vi "FLL Tournament Display.vi"() -> ()   [LabVIEW 2013]
uses:
  Team_List_Ctrl.ctl
  Team_Scores_And_Rankings_Array_Ctrl.ctl
  Round_And_Score_Ctrl.ctl
  Timer_Details_Ctrl.ctl
  <vilib>/httpClient/LabVIEWHTTPClient.lvlib
panel:
  out "Cancelled?":bool
  out "IP Address / Port":string
  in  "Scores Tab":enum32{"Page 1"}(tab)
  in  "Scores Box":i32(listbox)=3
  in  "Top Tab":enum32{"Page 1"}(tab)
  out "Main Logo Image":picture
  out "Powered By LabVIEW":picture
  out "FIRST LEGO League":picture
  out "Match Indicator":string
  out "Tournament Title String":string="2013 FIRST LEGO League Nature's Fury"
  out "TIMER":string="2 : 3 0"
  out "Top Sponsor Image":picture
  out "Mid Sponsor Image":picture
  out "Bottom Sponsor Image":picture
  out "Timer Properties":T1
  out "Consolidated Scores and Rankings":T3(array[cluster])
  out "Reported Scores and Rankings":T4
  out "Full Team List":T5[](array[typedef])
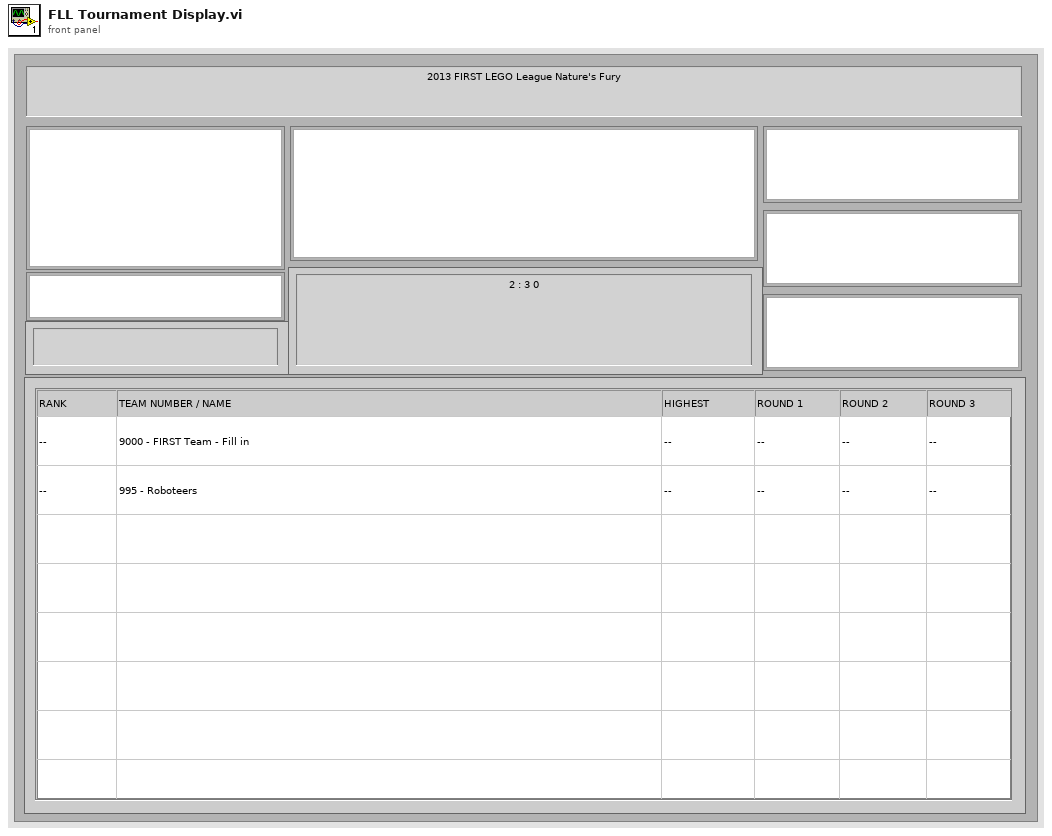
[diagram p1: front panel]
types:
  T1 = typedef "Timer_Details_Ctrl.ctl" = cluster{"TimeRemaining":string, "MatchPhase":string, "CurrentMatch":string, "Timer_Running":string}
  T2 = typedef "Round_And_Score_Ctrl.ctl" = cluster{"Score":string, "Round Number":string}
  T3 = cluster{"Rank":string, "Team Number":string, "Team Name":string, "Highest Score":string, "Scores":T2[]}[]
  T4 = typedef "Team_Scores_And_Rankings_Array_Ctrl.ctl" = cluster{"Rank":string, "Team Number":string, "Team Name":string, "Highest Score":string, "Scores":T2[]}[]
  T5 = typedef "Team_List_Ctrl.ctl" = cluster{"Team Name":string, "Team Number":string}
  T6 = typedef "LabVIEWHTTPClient.lvlib/ClientHandle.ctl" = refnum<k1>
  T7 = typedef "Team_List_Array_Ctrl.ctl" = T5[]
  T8 = cluster{"[0]":string, "[1]":string, "[2]":string, "[3]":string}
  T9 = enum32{"Invalid", "Standard", "Closed", "Hidden", "Minimized", "Maximized"}
  T10 = enum32{"invalid app kind", "Development System", "Run Time System", "Student Edition", "Embedded LabVIEW", "Evaluation", "Custom"}
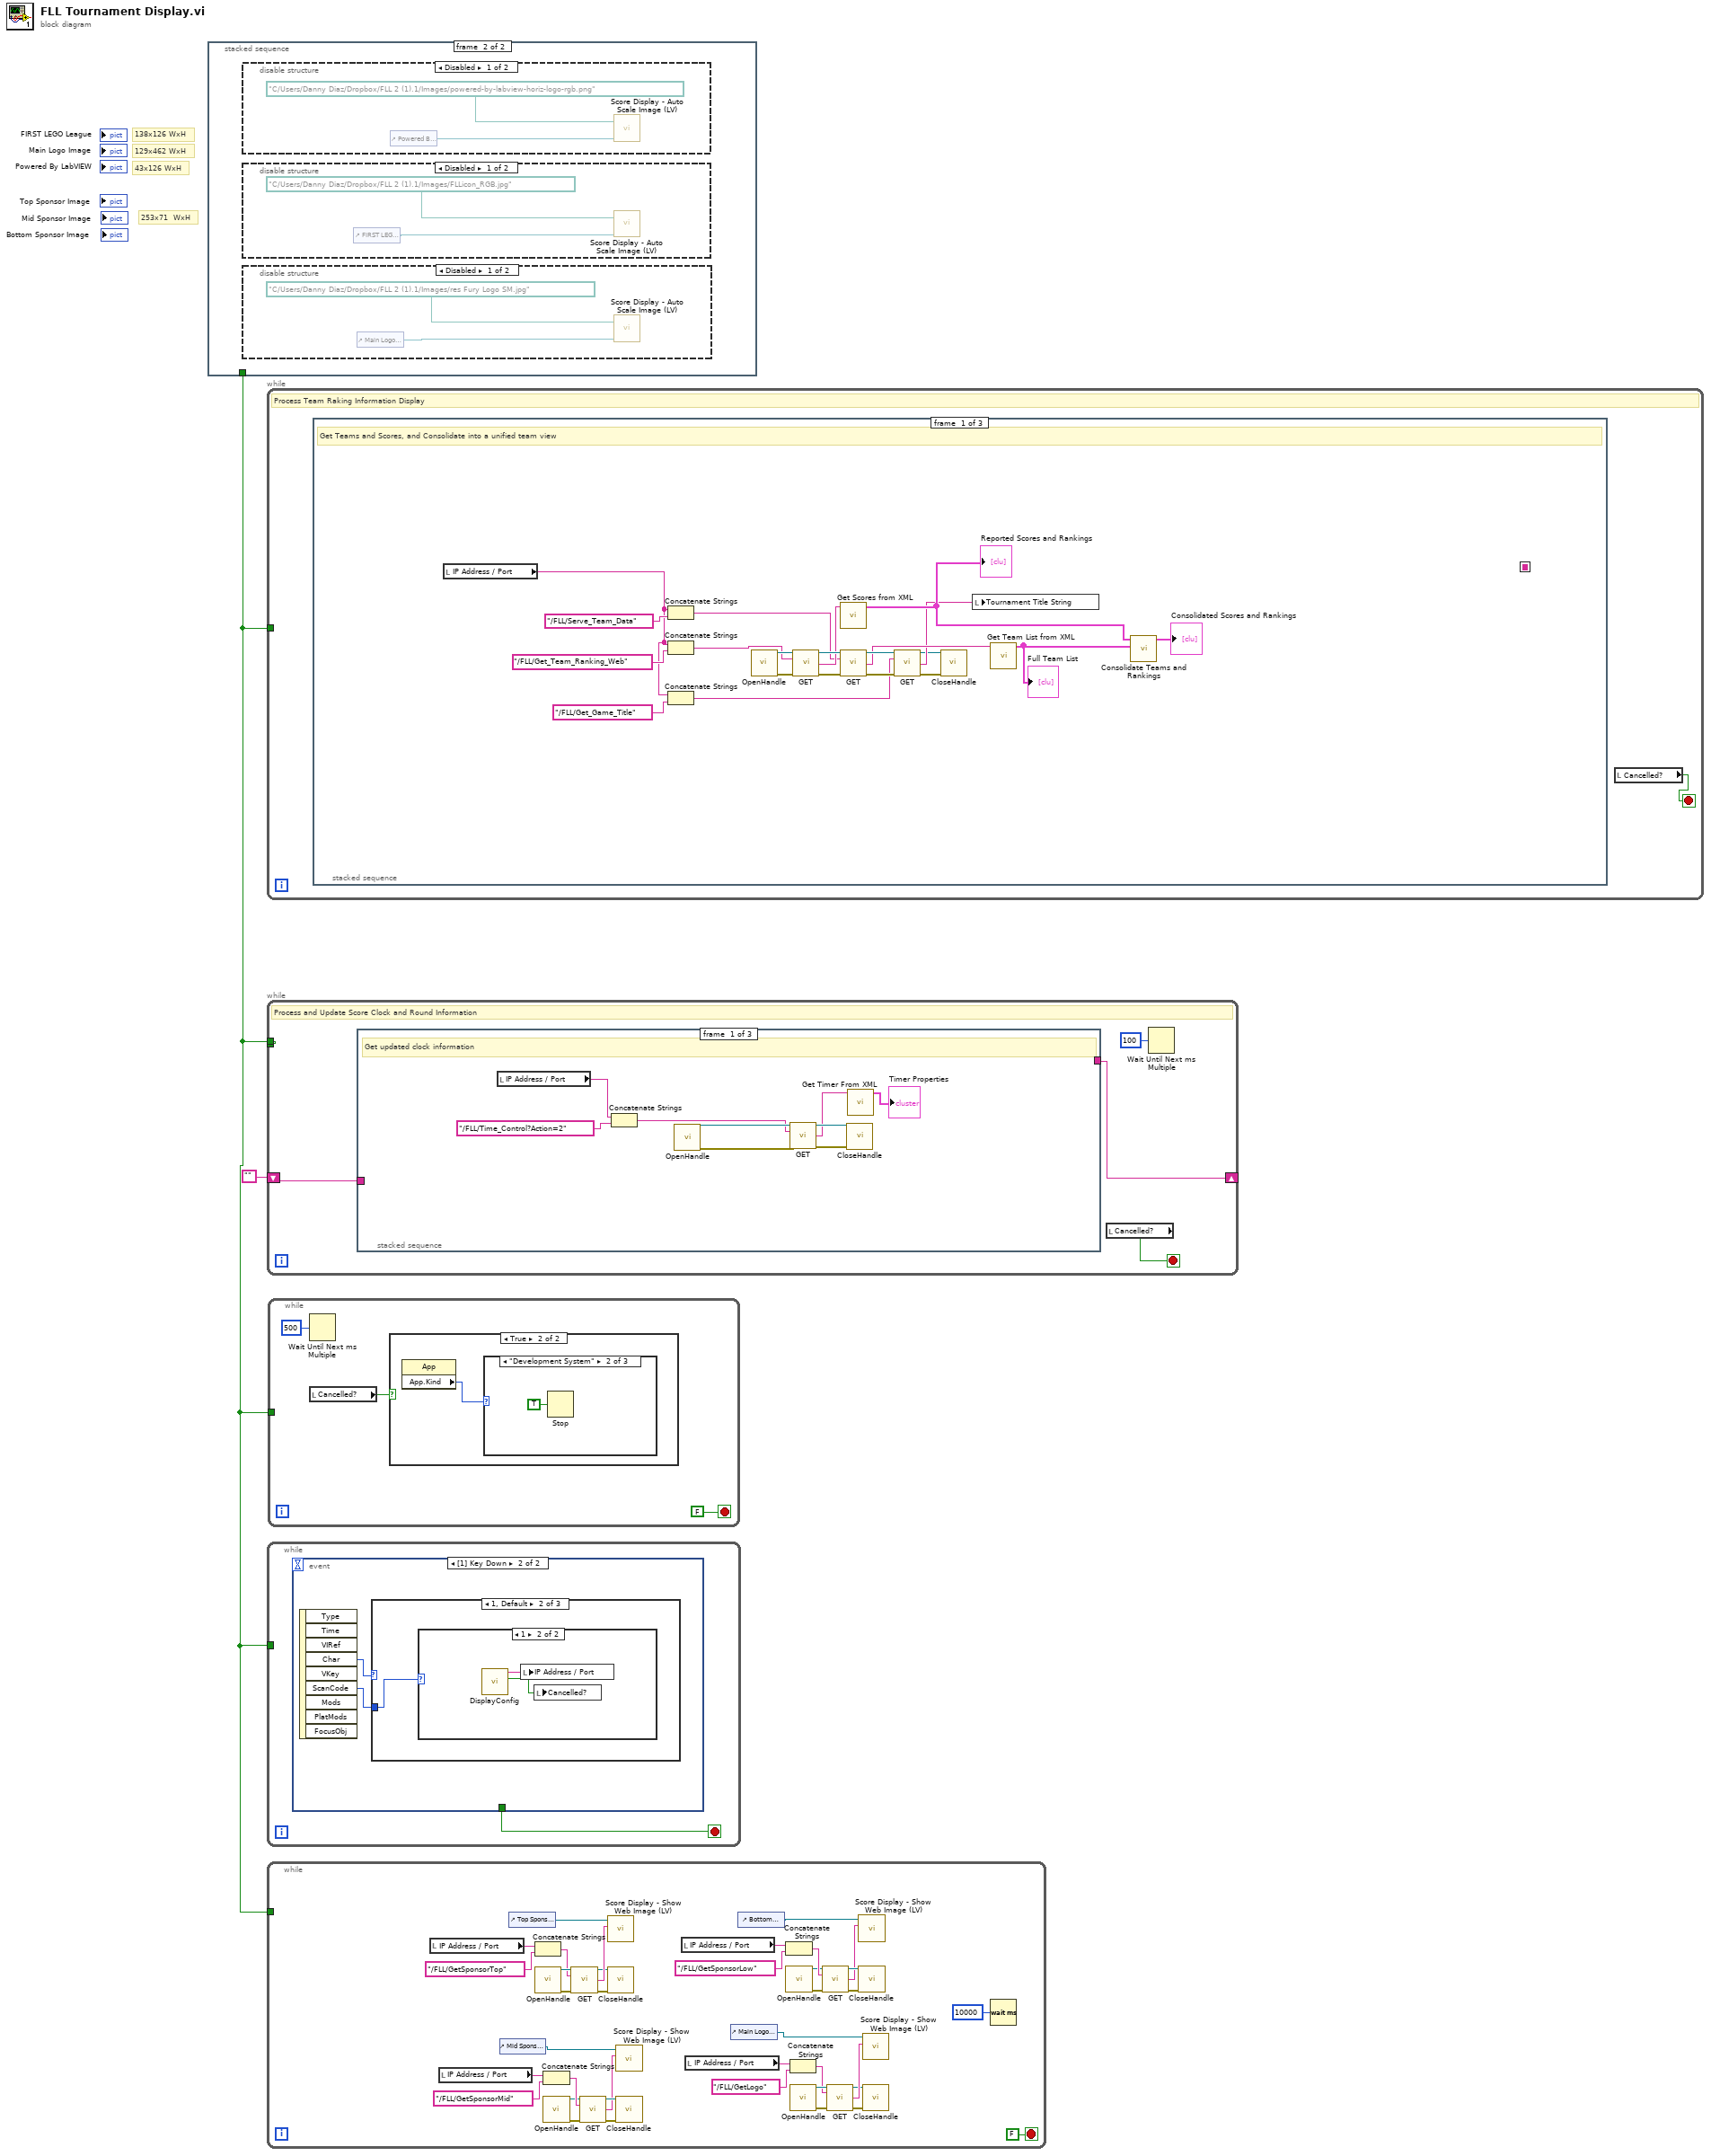
[diagram p0: block diagram]
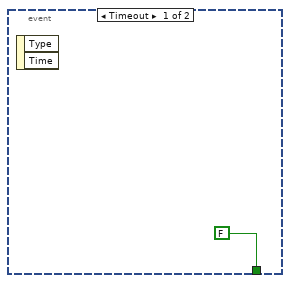
[diagram p2: hidden frame]
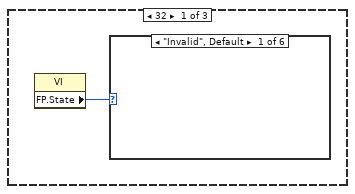
[diagram p3: hidden frame]
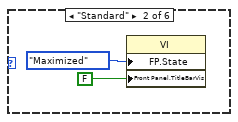
[diagram p4: hidden frame]
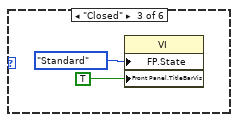
[diagram p5: hidden frame]
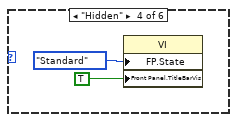
[diagram p6: hidden frame]
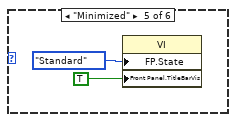
[diagram p7: hidden frame]
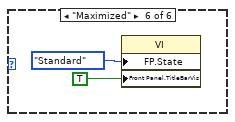
[diagram p8: hidden frame]
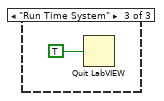
[diagram p13: hidden frame]
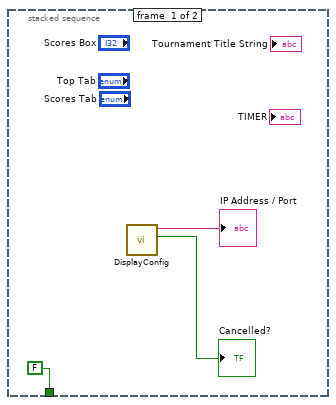
[diagram p14: hidden frame]
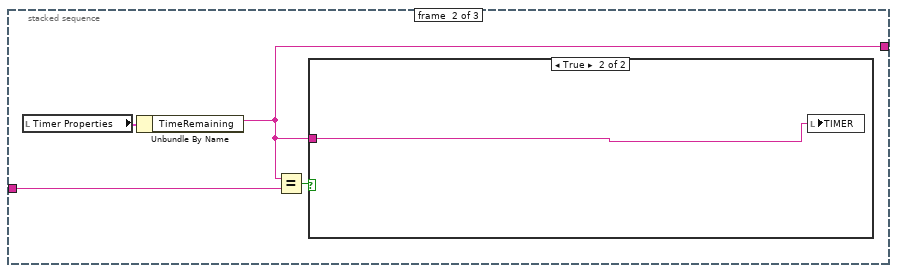
[diagram p18: hidden frame]
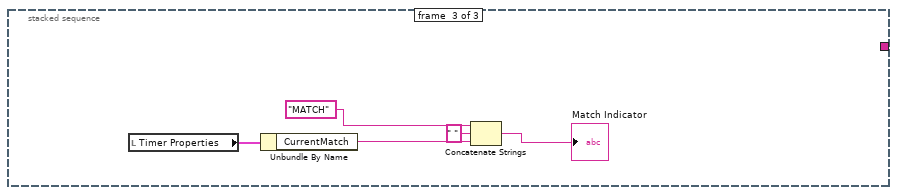
[diagram p20: hidden frame]
diagram:
  # "129x462 WxH"
  # "43x126 WxH"
  # "253x71  WxH"
  # "138x126 WxH"
  n1 = stacked-sequence {
    tunnel: [FALSE _] -> w1
    frame #0 {
      n2 = call "DisplayConfig.vi"() -> ("Cancelled?"=→"Cancelled?":bool, "String"=→"IP Address / Port":string)  [unwired: 10 in]
    }
    frame #1 {
      n3 = disable-structure shown="Disabled" {
        frame Disabled {
          n4 = control-ref of="Powered By LabVIEW"() -> (w10:refnum<vi>)
          n5 = call "Score Display - Auto Scale Image (LV).vi"("Picture Reference"=w10, "path to image file"=path "C:/Users/Danny Diaz/Dropbox/FLL 2 (1).1/Images/powered-by-labview-horiz-logo-rgb.png") -> ()  [unwired: 1 out]
        }
        frame Enabled {
        }
      }
      n6 = disable-structure shown="Disabled" {
        frame Disabled {
          n7 = control-ref of="FIRST LEGO League"() -> (w8:refnum<vi>)
          n8 = call "Score Display - Auto Scale Image (LV).vi"("Picture Reference"=w8, "path to image file"=path "C:/Users/Danny Diaz/Dropbox/FLL 2 (1).1/Images/FLLicon_RGB.jpg") -> ()  [unwired: 1 out]
        }
        frame Enabled {
        }
      }
      n9 = disable-structure shown="Disabled" {
        frame Disabled {
          n10 = control-ref of="Main Logo Image"() -> (w6:refnum<vi>)
          n11 = call "Score Display - Auto Scale Image (LV).vi"("Picture Reference"=w6, "path to image file"=path "C:/Users/Danny Diaz/Dropbox/FLL 2 (1).1/Images/res Fury Logo SM.jpg") -> ()  [unwired: 1 out]
        }
        frame Enabled {
        }
      }
    }
  }
  n12 = while {
    tunnel: w1 -> [_]
    stop <- w12 stop-if-true
    # "Process Team Raking Information Display"
    n13 = stacked-sequence {
      seq-local: [_ w34 _] -> [_ _ w85]
      frame #0 {
        # "Get Teams and Scores, and Consolidate into a unified team view"
        n14 = local read "IP Address / Port"() -> (w17:string)
        n15 = Concatenate Strings(w17, "/FLL/Serve_Team_Data" ("url")) -> (w24:string)
        n16 = Concatenate Strings(w17, "/FLL/Get_Team_Ranking_Web" ("url")) -> (w22:string)
        n17 = Concatenate Strings(w17, "/FLL/Get_Game_Title" ("url")) -> (w16:string)
        n18 = call <vilib>:"OpenHandle.vi"() -> ("client handle out"=w33:T6, "error out"=w31:errorcluster)  [unwired: 14 in]
        n19 = call <vilib>:"GET.vi"("client handle"=w33, "url"=w22, "error in (no error)"=w31) -> ("client handle out"=w30:T6, "body"=w29:string, "error out"=w32:errorcluster)  [unwired: 9 in, 1 out]
        n20 = call "Get Scores from XML.vi"("XML In"=w29) -> ("Team_Scores_And_Rankings_Array"=w27:T3)  [unwired: 9 in, 1 out]
        "Reported Scores and Rankings" <- w27
        n21 = call <vilib>:"GET.vi"("client handle"=w30, "url"=w24, "error in (no error)"=w32) -> ("client handle out"=w21:T6, "body"=w19:string, "error out"=w20:errorcluster)  [unwired: 9 in, 1 out]
        n22 = call <vilib>:"GET.vi"("client handle"=w21, "url"=w16, "error in (no error)"=w20) -> ("client handle out"=w14:T6, "body"=w15:string, "error out"=w13:errorcluster)  [unwired: 9 in, 1 out]
        n23 = call <vilib>:"CloseHandle.vi"("client handle"=w14, "error in (no error)"=w13) -> ()  [unwired: 13 in, 1 out]
        n24 = local write "Tournament Title String"(w15) -> ()
        n25 = call "Get Team List from XML.vi"("XML In"=w19) -> ("Team List Array"=w28:T7)  [unwired: 10 in]
        "Full Team List" <- w28
        n26 = call "Consolidate Teams and Rankings.vi"("Team List Array"=w28, "Team_Scores_And_Rankings_Array"=w27) -> ("Consolidated Teams and Rankings"=→"Consolidated Scores and Rankings":T3)  [unwired: 9 in]
      }
      frame #1 {
        n27 = local read "Consolidated Scores and Rankings"() -> (w37:T3)
        n28 = for {
          tunnel: w37 -> [w48] mode=indexing
          tunnel: [w47] -> w35 mode=indexing
          n29 = Unbundle By Name(w48) -> ("Rank"=w50:string, "Team Number"=w42:string, "Team Name"=w41:string, "Highest Score"=w46:string, "Scores"=w58:T2[])
          n30 = case shown="\"False\", Default" w50 {
            selector: w50 -> [w70 _]
            tunnel: [w69 1000] -> w49
            frame "False", Default {
              n31 = Decimal String To Number(string=w70) -> (number=w69:i32)  [unwired: 2 in, 1 out]
            }
            frame "--" {
            }
          }
          n32 = for {
            N: 4 -> [_]
            tunnel: w58 -> [w74]
            tunnel: [w72] -> w44 mode=indexing
            i -> [w75]
            n33 = Increment(x=w75) -> (x+1=w73:i32)
            n34 = for {
              tunnel: w74 -> [w77] mode=indexing
              tunnel: w73 -> [w81]
              tunnel: [w76] -> w72
              stop <- w78 stop-if-true
              n35 = Unbundle By Name(w77) -> ("Round Number"=w80:string, "Score"=w76:string)
              n36 = Number To Decimal String(number=w81) -> (decimal integer string=w79:string)  [unwired: 1 in]
              n37 = Equal?(x=w79, y=w80) -> (x = y?=w78:bool)
            }
          }
          n38 = case shown="\"False\", Default" w46 {
            selector: w46 -> [w65 w68]
            tunnel: [w66 w68] -> w45
            frame "False", Default {
              n39 = Decimal String To Number(string=w65) -> (number=w67:i32)  [unwired: 2 in, 1 out]
              n40 = Number To Decimal String(number=w67) -> (decimal integer string=w66:string)  [unwired: 1 in]
            }
            frame "--" {
            }
          }
          n41 = for {
            tunnel: w44 -> [w60] mode=indexing
            tunnel: [w59] -> w43 mode=indexing
            n42 = case shown="\"False\", Default" w60 {
              selector: w60 -> [w61 w64]
              tunnel: [w62 w64] -> w59
              frame "False", Default {
                n43 = Decimal String To Number(string=w61) -> (number=w63:i32)  [unwired: 2 in, 1 out]
                n44 = Number To Decimal String(number=w63) -> (decimal integer string=w62:string)  [unwired: 1 in]
              }
              frame "--" {
              }
            }
          }
          n45 = call "Build Text"("team_number"=w42, "team_name"=w41) -> ("Result"=w40:string)  [unwired: 12 in, 1 out]
          n46 = Array To Cluster(array=w43) -> (cluster=w56:T8)
          n47 = Unbundle(w56) -> ("[0]"=w55:string, "[1]"=w54:string, "[2]"=w53:string, "[3]"=w52:string)
          n48 = Build Array(w50, w40, w45, w55, w54, w53, w52) -> (w51:string[])
          n49 = Bundle(w49, w51) -> (w47:cluster{i32, string[]})  [unwired: 1 in]
        }
        n50 = Sort 1D Array(array=w35) -> (sorted array=w36:cluster{i32, string[]}[])
        n51 = for {
          tunnel: w36 -> [w39] mode=indexing
          tunnel: [w38] -> w34 mode=indexing
          n52 = Unbundle(w39) -> (w38:string[])  [unwired: 1 out]
        }
      }
      frame #2 {
        n53 = Array Size(array=w85) -> (size(s)=w83:i32[])
        n54 = Index Array(array=w83, index=0) -> (element=w82:i32)
        n55 = Divide(x=w82, y=8.0) -> (x/y=w87:dbl)
        n56 = Round Toward +Infinity(x=w87) -> (ceil(x): smallest int >= x=w86:dbl)
        n57 = for {
          N: w86 -> [_]
          tunnel: w85 -> [w90]
          i -> [w89]
          n58 = stacked-sequence {
            tunnel: w90 -> [w95 _]
            tunnel: w89 -> [w94 _]
            frame #0 {
              w93 = 8 ("length")
              n59 = Multiply(x=w93, y=w94) -> (x*y=w92:i32)
              n60 = Array Subset(array=w95, index (row)=w92, length (row)=w93) -> (w91:string[][])  [unwired: 2 in]
              n61 = property on="Scores Box" class="MCListbox (strict)"("ItemNames"=w91) -> ()  [unwired: 2 in, 2 out]
            }
            frame #1 {
              n62 = Wait Until Next ms Multiple(millisecond multiple=u32 5000) -> ()  [unwired: 1 out]
            }
          }
        }
      }
    }
    n63 = local read "Cancelled?"() -> (w12:bool)
  }
  n64 = while {
    shift-right: [w99] -> _
    shift-left: "" -> [w100]
    tunnel: [w98] -> _
    tunnel: w1 -> [w98]
    stop <- w97 stop-if-true
    # "Process and Update Score Clock and Round Information"
    n65 = stacked-sequence {
      tunnel: w100 -> [_ w112 _]
      tunnel: [_ w111 _] -> w99
      frame #0 {
        # "Get updated clock information"
        n66 = local read "IP Address / Port"() -> (w104:string)
        n67 = Concatenate Strings(w104, "/FLL/Time_Control?Action=2" ("url")) -> (w102:string)
        n68 = call <vilib>:"OpenHandle.vi"() -> ("client handle out"=w109:T6, "error out"=w107:errorcluster)  [unwired: 14 in]
        n69 = call <vilib>:"GET.vi"("client handle"=w109, "url"=w102, "error in (no error)"=w107) -> ("client handle out"=w108:T6, "body"=w105:string, "error out"=w106:errorcluster)  [unwired: 9 in, 1 out]
        n70 = call <vilib>:"CloseHandle.vi"("client handle"=w108, "error in (no error)"=w106) -> ()  [unwired: 13 in, 1 out]
        n71 = call "Get Timer From XML.vi"("body"=w105) -> ("Cluster"=→"Timer Properties":T1)  [unwired: 9 in, 1 out]
      }
      frame #1 {
        n72 = local read "Timer Properties"() -> (w114:T1)
        n73 = Unbundle By Name(w114) -> ("TimeRemaining"=w111:string)
        n74 = Equal?(x=w111, y=w112) -> (x = y?=w113:bool)
        n75 = case shown="True" w113 {
          tunnel: w111 -> [_ w115]
          frame False {
          }
          frame True {
            n76 = local write "TIMER"(w115) -> ()
          }
        }
      }
      frame #2 {
        n77 = local read "Timer Properties"() -> (w120:T1)
        n78 = Unbundle By Name(w120) -> ("CurrentMatch"=w118:string)
        n79 = Concatenate Strings("MATCH", " " ("string"), w118) -> (→"Match Indicator":string)
      }
    }
    n80 = local read "Cancelled?"() -> (w97:bool)
    n81 = Wait Until Next ms Multiple(millisecond multiple=u32 100) -> ()  [unwired: 1 out]
  }
  n82 = while {
    tunnel: w1 -> [_]
    stop <- w121 stop-if-true
    n83 = event shown="[1] Key Down" {
      selector: _ -> [_ _]
      dyn-events: _ -> [_ _]
      timeout: _ -> [_ _]
      tunnel: [FALSE _] -> w121
      event Timeout {
        n84 = event-data() -> ()  [unwired: 1 in, 2 out]
      }
      event Key Down {
        n85 = event-data() -> ("Char"=w124:i16, "ScanCode"=w123:i16)  [unwired: 1 in, 7 out]
        n86 = case shown="1, Default" w124 {
          tunnel: w123 -> [_ w136 _]
          frame 32 {
            n87 = property class="VI"() -> ("FP.State"=w125:T9)  [unwired: 2 in, 2 out]
            n88 = case shown="\"Invalid\", Default" w125 {
              frame "Invalid", Default {
              }
              frame "Standard" {
                n89 = property class="VI"("FP.State"=T9."Maximized" ("Front Panel Window:State"), "Front Panel.TitleBarVis"=FALSE ("Front Panel Window:Title Bar Visible")) -> ()  [unwired: 2 in, 2 out]
              }
              frame "Closed" {
                n90 = property class="VI"("FP.State"=T9."Standard" ("Front Panel Window:State"), "Front Panel.TitleBarVis"=TRUE ("Front Panel Window:Title Bar Visible")) -> ()  [unwired: 2 in, 2 out]
              }
              frame "Hidden" {
                n91 = property class="VI"("FP.State"=T9."Standard" ("Front Panel Window:State"), "Front Panel.TitleBarVis"=TRUE ("Front Panel Window:Title Bar Visible")) -> ()  [unwired: 2 in, 2 out]
              }
              frame "Minimized" {
                n92 = property class="VI"("FP.State"=T9."Standard" ("Front Panel Window:State"), "Front Panel.TitleBarVis"=TRUE ("Front Panel Window:Title Bar Visible")) -> ()  [unwired: 2 in, 2 out]
              }
              frame "Maximized" {
                n93 = property class="VI"("FP.State"=T9."Standard" ("Front Panel Window:State"), "Front Panel.TitleBarVis"=TRUE ("Front Panel Window:Title Bar Visible")) -> ()  [unwired: 2 in, 2 out]
              }
            }
          }
          frame 1, Default {
            n94 = case shown="1" w136 {
              frame 0, Default {
              }
              frame 1 {
                n95 = call "DisplayConfig.vi"() -> ("Cancelled?"=w138:bool, "String"=w137:string)  [unwired: 10 in]
                n96 = local write "IP Address / Port"(w137) -> ()
                n97 = local write "Cancelled?"(w138) -> ()
              }
            }
          }
          frame 27 {
            # "Pressed C"
          }
        }
      }
    }
  }
  n98 = while {
    tunnel: w1 -> [_]
    stop <- FALSE stop-if-true
    n99 = local read "IP Address / Port"() -> (w158:string)
    n100 = local read "IP Address / Port"() -> (w176:string)
    n101 = control-ref of="Mid Sponsor Image"() -> (w149:refnum<vi>)
    n102 = control-ref of="Top Sponsor Image"() -> (w165:refnum<vi>)
    n103 = Concatenate Strings(w158, "/FLL/GetSponsorTop" ("url")) -> (w159:string)
    n104 = call <vilib>:"OpenHandle.vi"() -> ("client handle out"=w163:T6, "error out"=w164:errorcluster)  [unwired: 14 in]
    n105 = Concatenate Strings(w176, "/FLL/GetSponsorMid" ("url")) -> (w175:string)
    n106 = call <vilib>:"OpenHandle.vi"() -> ("client handle out"=w171:T6, "error out"=w170:errorcluster)  [unwired: 14 in]
    n107 = call <vilib>:"GET.vi"("client handle"=w163, "url"=w159, "error in (no error)"=w164) -> ("client handle out"=w162:T6, "body"=w166:string, "error out"=w161:errorcluster)  [unwired: 9 in, 1 out]
    n108 = call <vilib>:"GET.vi"("client handle"=w171, "url"=w175, "error in (no error)"=w170) -> ("client handle out"=w172:T6, "body"=w167:string, "error out"=w173:errorcluster)  [unwired: 9 in, 1 out]
    n109 = call "Score Display - Show Web Image (LV).vi"("body"=w166, "Picture in"=w165) -> ()  [unwired: 10 in]
    n110 = call <vilib>:"CloseHandle.vi"("client handle"=w162, "error in (no error)"=w161) -> ()  [unwired: 13 in, 1 out]
    n111 = call "Score Display - Show Web Image (LV).vi"("body"=w167, "Picture in"=w149) -> ()  [unwired: 10 in]
    n112 = call <vilib>:"CloseHandle.vi"("client handle"=w172, "error in (no error)"=w173) -> ()  [unwired: 13 in, 1 out]
    n113 = local read "IP Address / Port"() -> (w157:string)
    n114 = local read "IP Address / Port"() -> (w140:string)
    n115 = control-ref of="Main Logo Image"() -> (w139:refnum<vi>)
    n116 = control-ref of="Bottom Sponsor Image"() -> (w148:refnum<vi>)
    n117 = Concatenate Strings(w157, "/FLL/GetSponsorLow" ("url")) -> (w156:string)
    n118 = call <vilib>:"OpenHandle.vi"() -> ("client handle out"=w152:T6, "error out"=w151:errorcluster)  [unwired: 14 in]
    n119 = Concatenate Strings(w140, "/FLL/GetLogo" ("url")) -> (w141:string)
    n120 = call <vilib>:"OpenHandle.vi"() -> ("client handle out"=w145:T6, "error out"=w146:errorcluster)  [unwired: 14 in]
    n121 = call <vilib>:"GET.vi"("client handle"=w152, "url"=w156, "error in (no error)"=w151) -> ("client handle out"=w153:T6, "body"=w150:string, "error out"=w154:errorcluster)  [unwired: 9 in, 1 out]
    n122 = call <vilib>:"GET.vi"("client handle"=w145, "url"=w141, "error in (no error)"=w146) -> ("client handle out"=w144:T6, "body"=w147:string, "error out"=w143:errorcluster)  [unwired: 9 in, 1 out]
    n123 = call "Score Display - Show Web Image (LV).vi"("body"=w150, "Picture in"=w148) -> ()  [unwired: 10 in]
    n124 = call <vilib>:"CloseHandle.vi"("client handle"=w153, "error in (no error)"=w154) -> ()  [unwired: 13 in, 1 out]
    n125 = call "Score Display - Show Web Image (LV).vi"("body"=w147, "Picture in"=w139) -> ()  [unwired: 10 in]
    n126 = call <vilib>:"CloseHandle.vi"("client handle"=w144, "error in (no error)"=w143) -> ()  [unwired: 13 in, 1 out]
    n127 = Wait (ms)(milliseconds to wait=u32 10000) -> ()  [unwired: 1 out]
  }
  n128 = while {
    tunnel: w1 -> [_]
    stop <- FALSE stop-if-true
    n129 = Wait Until Next ms Multiple(millisecond multiple=u32 500) -> ()  [unwired: 1 out]
    n130 = local read "Cancelled?"() -> (w179:bool)
    n131 = case shown="True" w179 {
      frame False {
      }
      frame True {
        n132 = property class="App"() -> ("App.Kind"=w180:T10)  [unwired: 2 in, 2 out]
        n133 = case shown="\"Development System\"" w180 {
          frame "invalid app kind", Default {
          }
          frame "Development System" {
            n134 = Stop(stop? (T)=TRUE) -> ()
          }
          frame "Run Time System" {
            n135 = Quit LabVIEW(quit? (T)=TRUE ("stop? (T)")) -> ()
          }
        }
      }
    }
  }
